vi "Get Default Report Path.vi"(10 "File Extension":string="xml") -> (2 "Default Report Directory":path, 3 "Default Report Path":path)   [LabVIEW 2020, in "Paths.lvlib"]
uses:
  Paths.lvlib
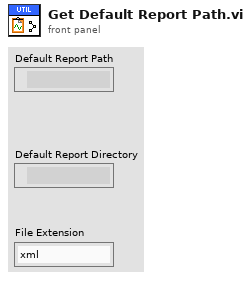
[diagram p1: front panel]
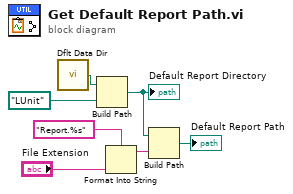
[diagram p0: block diagram]
diagram:
  n1 = call <vilib>:"Dflt Data Dir.vi"() -> ("App:Default Data Directory"=w6:path)
  n2 = Build Path(base path=w6, name or relative path=path "LUnit") -> (appended path=w4:path)
  "Default Report Directory" <- w4
  n3 = Format Into String(format string="Report.%s", "File Extension") -> (resulting string=w1:string)  [unwired: 2 in, 1 out]
  n4 = Build Path(base path=w4, name or relative path=w1) -> (appended path=→"Default Report Path":path)
